vi "Read Waveform from TDMS (Scaled and Reduced Resolution).vi"(0 "VISA resource name":refnum<visa-resource-name>, 1 "Start Point (0)":i32, 2 "TDMS Path":path, 5 "Measurement Source (1: Channel 1)":i32(ring)=1 items=["Channel 1"=1, "Channel 2"=2, "Channel 3"=3, "Channel 4"=4, "Function 1"=5, "Function 2"=6, "Function 3"=7, "Function 4"=8, "Memory 1"=9, "Memory 2"=10, "Memory 3"=11, "Memory 4"=12], 7 "Length (1000)":i32=10000 caption="Length (10000)", 9 "Waveform Size (100)":i32=1000 caption="Waveform Size (1000)", 11 "error in (no error)":errorcluster) -> (4 "VISA resource name out":refnum<visa-resource-name>, 6 "Waveform Information":T1, 8 "Waveform Data":waveform(dbl)(graph), 15 "error out":errorcluster)   [LabVIEW 2020, in "Agilent 90000 Series.lvlib"]
doc: "Returns a decimated and scaled waveform. The points will be read from TDMS in chunks and a Min/Max decimating is performed on them."
uses:
  Agilent 90000 Series.lvlib
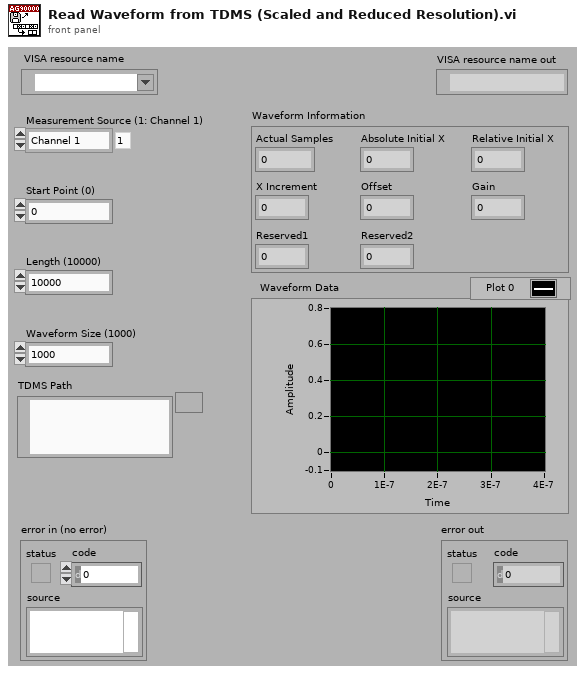
[diagram p1: front panel]
types:
  T1 = cluster{"Actual Samples":i32, "Absolute Initial X":dbl, "Relative Initial X":dbl, "X Increment":dbl, "Offset":dbl, "Gain":dbl, "Reserved1":dbl, "Reserved2":dbl}
  T2 = enum16{"open", "open or create", "create or replace", "create", "open (read-only)"}
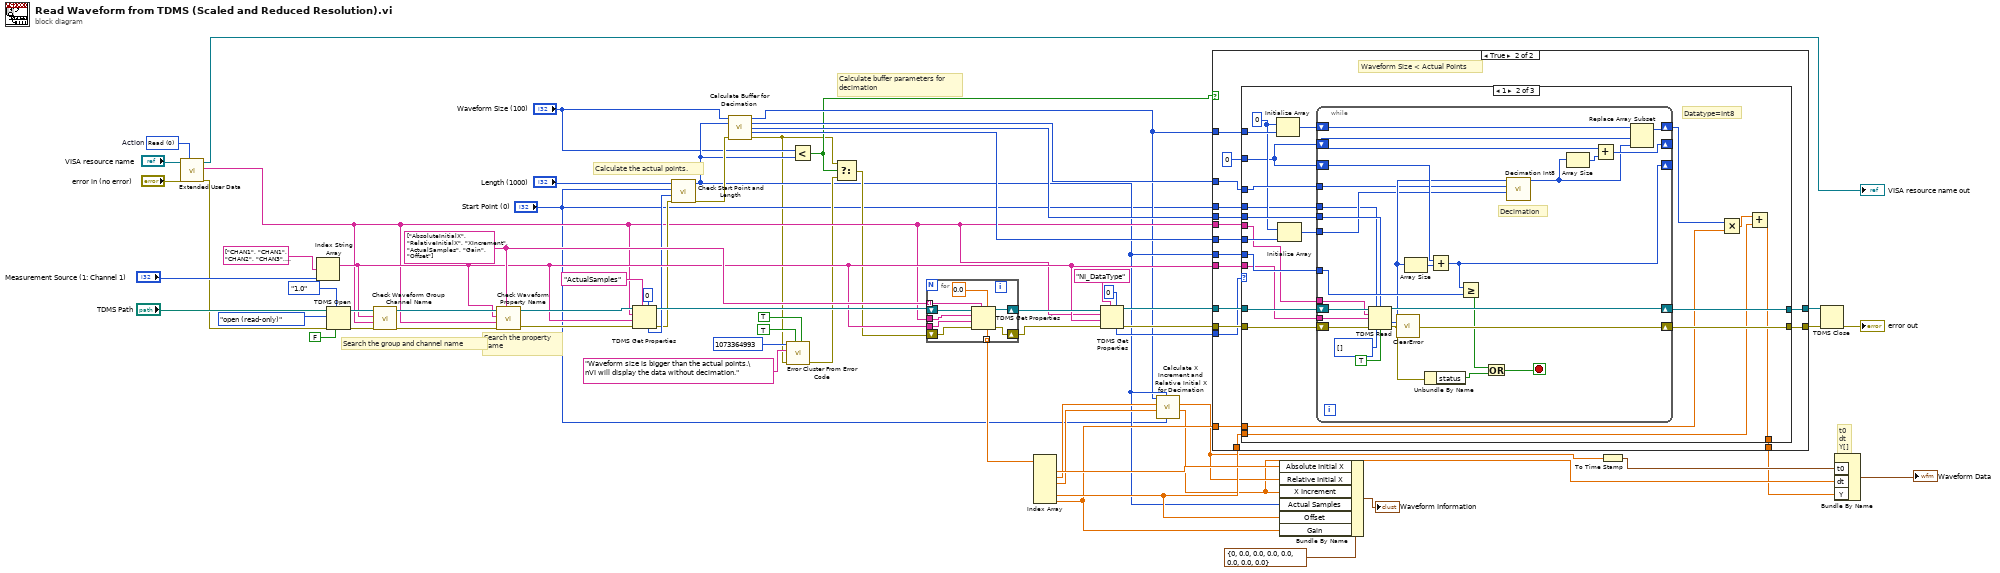
[diagram p0: block diagram]
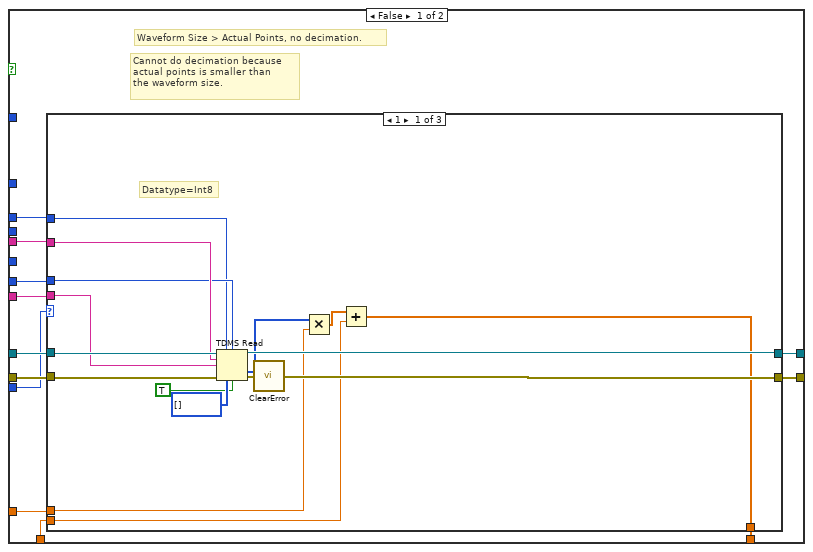
[diagram p2: hidden frame]
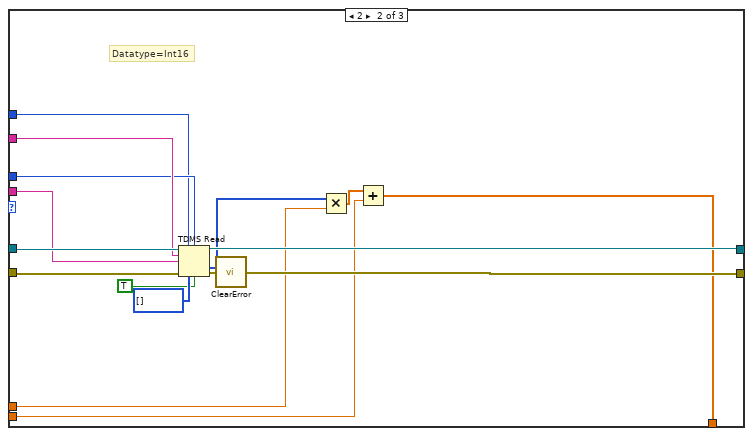
[diagram p3: hidden frame]
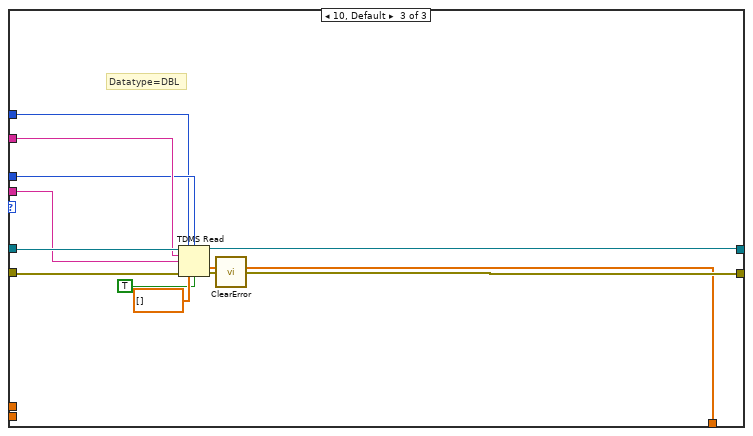
[diagram p4: hidden frame]
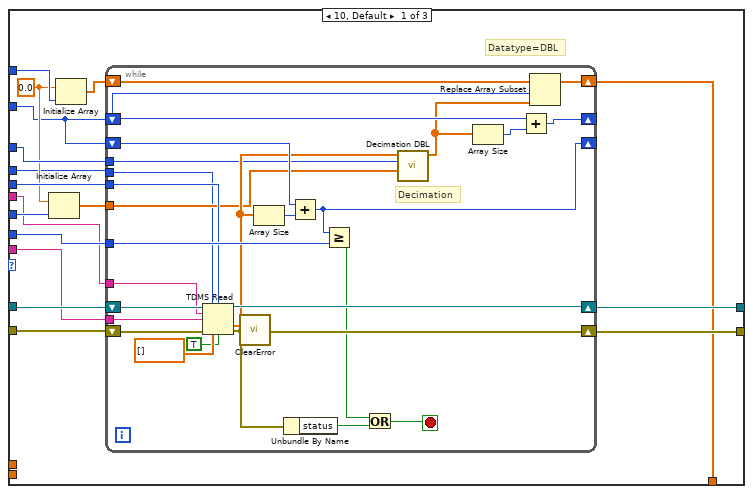
[diagram p5: hidden frame]
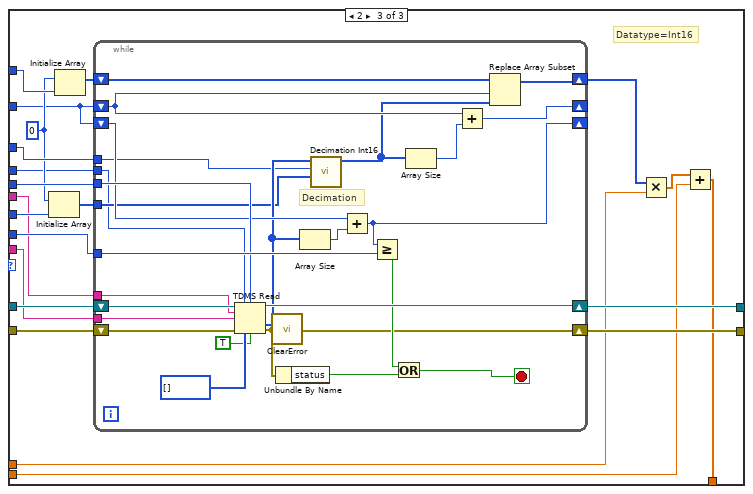
[diagram p6: hidden frame]
diagram:
  w26 = u16 0 items=["Read", "Write"]  # Action
  w57 = string[] ["AbsoluteInitialX", "RelativeInitialX", "XIncrement", "ActualSamples", "Gain", "Offset"] ("property names")
  # "t0\ndt\nY[]"
  # "Calculate buffer parameters for\ndecimation"
  # "Calculate the actual points."
  # "Search the property\nname"
  # "Search the group and channel name"
  n1 = call "Extended User Data.vi"("Action"=w26, "Error In (no error)"="error in (no error)", "VISA resource name in"="VISA resource name") -> ("Error Out"=w24:errorcluster, "Default Group Name Out"=w25:string, "VISA resource name out"=→"VISA resource name out":refnum<visa-resource-name>)  [unwired: 1 in, 5 out]
  n2 = Index String Array(1:"Measurement Source (1: Channel 1)", 2:string[] ["CHAN1", "CHAN1", "CHAN2", "CHAN3", "CHAN4", "FUNC1", "FUNC2", "FUNC3", "FUNC4", "WMEM1", "WMEM2", "WMEM3", "WMEM4"] ("subarray 2")) -> (0:w36:string)  [unwired: 1 out]
  n3 = TDMS Open(6:FALSE ("disable buffering? (T)"), 7:enum16{"1.0", "2.0"}."1.0" ("file format version (2.0)"), 8:w24, 10:T2."open (read-only)" ("operation (0:open)"), 11:"TDMS Path") -> (0:w55:errorcluster, 3:w56:refnum<k34>)  [unwired: 2 in]
  n4 = call "Check Waveform Group Channel Name.vi"("error in (no error)"=w55, "Group Name"=w25, "Channel Name"=w36, "TDMS File In"=w56) -> ("error out"=w54:errorcluster, "TDMS File Out"=w53:refnum<k34>)  [unwired: 6 out]
  n5 = call "Check Waveform Property Name.vi"("Property Name"=w57, "error in (no error)"=w54, "Group Name"=w25, "Channel Name"=w36, "TDMS File In"=w53) -> ("error out"=w50:errorcluster, "TDMS File Out"=w49:refnum<k34>)  [unwired: 5 out]
  n6 = TDMS Get Properties(5:0 ("Ring"), 7:"ActualSamples" ("property name"), 8:w50, 9:w36, 10:w25, 11:w49) -> (0:w31:errorcluster, 3:w46:refnum<k34>, 4:w32:i32)  [unwired: 3 out]
  n7 = call "Check Start Point and Length.vi"("error in (no error)"=w31, "Total Samples in TDMS (10000)"=w32, "Start Point (0)"="Start Point (0)", "Length (1000)"="Length (1000)") -> ("error out"=w30:errorcluster, "Actual Points"=w11:i32)  [unwired: 6 out]
  n8 = call "Calculate Buffer for Decimation.vi"("Waveform Size In (100)"="Waveform Size (100)", "Actual Points (1000)"=w11, "error in (no error)"=w30) -> ("Waveform Size Out"=w8:i32, "Number of Bytes per Chunck"=w10:i32, "Number of Bytes per Fetch"=w34:i32, "Decimation Buffer Size"=w33:i32, "error out"=w3:errorcluster)  [unwired: 1 in, 7 out]
  n9 = call <vilib>:"Error Cluster From Error Code.vi"("is warning? (False)"=TRUE, "show call chain? (False)"=TRUE, "error in (no error)"=w3, "error message (\"\")"="Waveform size is bigger than the actual points.\nVI will display the data without decimation." ("error message (\"\")"), "error code (0)"=1073364993) -> ("error out"=w20:errorcluster)  [unwired: 4 out]
  n10 = Less?(x="Waveform Size (100)", y=w11) -> (x < y?=w7:bool)
  n11 = Select(t=w3, s=w7, f=w20) -> (s? t:f=w19:errorcluster)
  n12 = for {
    tunnel: w36 -> [w71]
    tunnel: w25 -> [w70]
    shift-right: [w72] -> w42
    shift-left: w19 -> [w73]
    tunnel: w57 -> [w68] mode=indexing
    tunnel: [w66] -> w61 mode=indexing
    shift-right: [w69] -> w45
    shift-left: w46 -> [w74]
    n13 = TDMS Get Properties(5:0.0 ("Reserved1"), 7:w68, 8:w73, 9:w71, 10:w70, 11:w74) -> (0:w72:errorcluster, 3:w69:refnum<k34>, 4:w66:dbl)  [unwired: 3 out]
  }
  n14 = Index Array(array=w61) -> (element #1=w60:dbl, element #2=w18:dbl, element #3=w17:dbl, element #5=w40:dbl, element #6=w39:dbl)  [unwired: 6 in, 1 out]
  n15 = TDMS Get Properties(5:0 ("Ring"), 7:"NI_DataType" ("property name"), 8:w42, 9:w36, 10:w25, 11:w45) -> (0:w43:errorcluster, 3:w44:refnum<k34>, 4:w41:i32)  [unwired: 3 out]
  n16 = call "Calculate X Increment and Relative Initial X for Decimation.vi"("Start Point (0)"="Start Point (0)", "Actual Points (1000)"=w11, "Original X Increment (0)"=w17, "Original Relative Initial X (0)"=w18, "Waveform Size (100)"=w8) -> ("X Increment Out"=w13:dbl, "Relative Initial X Out"=w15:dbl)  [unwired: 5 out]
  n17 = case shown="True" w7 {
    tunnel: w44 -> [w86 w147]
    tunnel: w43 -> [w85 w146]
    tunnel: w41 -> [w84 w145]
    tunnel: w40 -> [w83 w144]
    tunnel: w39 -> [w82 w143]
    tunnel: [w81 w142] -> w38
    tunnel: [w80 w141] -> w37
    tunnel: w36 -> [w79 w140]
    tunnel: w34 -> [_ w139]
    tunnel: w33 -> [_ w138]
    tunnel: w25 -> [w78 w137]
    tunnel: [w77 w135] -> w5
    tunnel: w11 -> [w76 w134]
    tunnel: w10 -> [_ w133]
    tunnel: w8 -> [_ w132]
    tunnel: "Start Point (0)" -> [w75 w131]
    frame False {
      # "Cannot do decimation because\nactual points is smaller than \nthe waveform size."
      # "Waveform Size > Actual Points, no decimation."
      n18 = case shown="1" w84 {
        tunnel: w78 -> [w100 w116 w128]
        tunnel: w79 -> [w99 w115 w127]
        tunnel: w86 -> [w101 w117 w129]
        tunnel: w85 -> [w102 w118 w130]
        tunnel: w83 -> [w95 w111 _]
        tunnel: w82 -> [w96 w112 _]
        tunnel: w76 -> [w92 w108 w123]
        tunnel: [w98 w114 w126] -> w81
        tunnel: [w97 w113 w125] -> w80
        tunnel: [w89 w105 w121] -> w77
        tunnel: w75 -> [w91 w107 w122]
        frame 1 {
          # "Datatype=Int8"
          n19 = TDMS Read(0:w101, 1:w91, 2:w92, 5:w100, 7:w99, 11:w102, 12:i8[] [], 13:TRUE ("return channels in file order? (F)")) -> (4:w98:refnum<k34>, 10:w90:i8[], 15:w87:errorcluster)  [unwired: 3 out]
          n20 = call <vilib>:"ClearError.vi"("error in (no error)"=w87) -> ("error out"=w97:errorcluster)
          n21 = Multiply(x=w90, y=w96) -> (x*y=w94:dbl[])
          n22 = Add(x=w94, y=w95) -> (x+y=w89:dbl[])
        }
        frame 2 {
          # "Datatype=Int16"
          n23 = TDMS Read(0:w117, 1:w107, 2:w108, 5:w116, 7:w115, 11:w118, 12:i16[] [], 13:TRUE ("return channels in file order? (F)")) -> (4:w114:refnum<k34>, 10:w106:i16[], 15:w103:errorcluster)  [unwired: 3 out]
          n24 = call <vilib>:"ClearError.vi"("error in (no error)"=w103) -> ("error out"=w113:errorcluster)
          n25 = Multiply(x=w106, y=w112) -> (x*y=w110:dbl[])
          n26 = Add(x=w110, y=w111) -> (x+y=w105:dbl[])
        }
        frame 10, Default {
          # "Datatype=DBL"
          n27 = TDMS Read(0:w129, 1:w122, 2:w123, 5:w128, 7:w127, 11:w130, 12:dbl[] [], 13:TRUE ("return channels in file order? (F)")) -> (4:w126:refnum<k34>, 10:w121:dbl[], 15:w119:errorcluster)  [unwired: 3 out]
          n28 = call <vilib>:"ClearError.vi"("error in (no error)"=w119) -> ("error out"=w125:errorcluster)
        }
      }
    }
    frame True {
      # "Waveform Size < Actual Points"
      n29 = case shown="1" w145 {
        tunnel: w137 -> [w154 w202 w250]
        tunnel: w140 -> [w153 w201 w249]
        tunnel: w147 -> [w155 w203 w251]
        tunnel: w146 -> [w156 w204 w252]
        tunnel: w144 -> [_ w194 w242]
        tunnel: w143 -> [_ w197 w245]
        tunnel: w132 -> [w164 w212 w260]
        tunnel: 0 ("element") -> [w149 w195 w243]
        tunnel: w133 -> [w162 w210 w258]
        tunnel: w139 -> [w161 w209 w257]
        tunnel: w138 -> [w159 w207 w255]
        tunnel: w134 -> [w157 w205 w253]
        tunnel: [w152 w200 w248] -> w142
        tunnel: [w151 w199 w247] -> w141
        tunnel: [w150 w196 w244] -> w135
        tunnel: w131 -> [w148 w192 w240]
        frame 10, Default {
          w160 = 0.0 ("element")
          # "Datatype=DBL"
          n30 = Initialize Array(w160, w159) -> (w158:dbl[])
          n31 = Initialize Array(w160, w164) -> (w163:dbl[])
          n32 = while {
            shift-right: [w175] -> w151
            shift-left: w156 -> [w182]
            shift-right: [w191] -> w152
            shift-left: w155 -> [w190]
            shift-right: [w189] -> w150
            shift-left: w163 -> [w187]
            shift-right: [w188] -> _
            shift-left: w149 -> [w176]
            tunnel: w157 -> [w186]
            tunnel: w161 -> [w179]
            tunnel: w162 -> [w170]
            tunnel: w158 -> [w169]
            shift-right: [w183] -> _
            shift-left: w149 -> [w185]
            tunnel: w154 -> [w178]
            tunnel: w153 -> [w177]
            tunnel: w148 -> [w167]
            stop <- w172 stop-if-true
            # "Decimation"
            n33 = TDMS Read(0:w190, 1:w167, 2:w179, 5:w178, 7:w177, 11:w182, 12:dbl[] [], 13:TRUE ("return channels in file order? (F)")) -> (4:w191:refnum<k34>, 10:w171:dbl[], 15:w165:errorcluster)  [unwired: 3 out]
            n34 = call <vilib>:"ClearError.vi"("error in (no error)"=w165) -> ("error out"=w175:errorcluster)
            n35 = Array Size(array=w171) -> (size(s)=w180:i32)
            n36 = Unbundle By Name(w175) -> ("status"=w174:bool)
            n37 = Add(x=w176, y=w180) -> (x+y=w188:i32)
            n38 = Greater Or Equal?(x=w188, y=w186) -> (x >= y?=w173:bool)
            n39 = Or(x=w173, y=w174) -> (x .or. y?=w172:bool)
            n40 = call "Decimation DBL.vi"("Decimation Array"=w169, "Number of Bytes per Chunck (1000)"=w170, "Raw Data"=w171) -> ("Decimation Data"=w168:dbl[])  [unwired: 8 out]
            n41 = Array Size(array=w168) -> (size(s)=w184:i32)
            n42 = Add(x=w185, y=w184) -> (x+y=w183:i32)
            n43 = Replace Array Subset(array=w187, new element=w168, index=w185) -> (w189:dbl[])
          }
        }
        frame 1 {
          w208 = i8 0 ("element")
          # "Datatype=Int8"
          n44 = Initialize Array(w208, w212) -> (w211:i8[])
          n45 = Initialize Array(w208, w207) -> (w206:i8[])
          n46 = while {
            shift-right: [w222] -> w199
            shift-left: w204 -> [w230]
            shift-right: [w239] -> w200
            shift-left: w203 -> [w238]
            shift-right: [w237] -> w198
            shift-left: w211 -> [w235]
            shift-right: [w236] -> _
            shift-left: w195 -> [w224]
            tunnel: w205 -> [w234]
            tunnel: w209 -> [w227]
            tunnel: w210 -> [w218]
            tunnel: w206 -> [w217]
            shift-right: [w231] -> _
            shift-left: w195 -> [w233]
            tunnel: w202 -> [w226]
            tunnel: w201 -> [w225]
            tunnel: w192 -> [w215]
            stop <- w220 stop-if-true
            # "Decimation"
            n47 = TDMS Read(0:w238, 1:w215, 2:w227, 5:w226, 7:w225, 11:w230, 12:i8[] [], 13:TRUE ("return channels in file order? (F)")) -> (4:w239:refnum<k34>, 10:w219:i8[], 15:w213:errorcluster)  [unwired: 3 out]
            n48 = call <vilib>:"ClearError.vi"("error in (no error)"=w213) -> ("error out"=w222:errorcluster)
            n49 = Array Size(array=w219) -> (size(s)=w228:i32)
            n50 = Unbundle By Name(w222) -> ("status"=w223:bool)
            n51 = Add(x=w224, y=w228) -> (x+y=w236:i32)
            n52 = Greater Or Equal?(x=w236, y=w234) -> (x >= y?=w221:bool)
            n53 = Or(x=w221, y=w223) -> (x .or. y?=w220:bool)
            n54 = call "Decimation Int8.vi"("Decimation Array"=w217, "Number of Bytes per Chunck (1000)"=w218, "Raw Data"=w219) -> ("Decimation Data"=w216:i8[])  [unwired: 8 out]
            n55 = Array Size(array=w216) -> (size(s)=w232:i32)
            n56 = Add(x=w233, y=w232) -> (x+y=w231:i32)
            n57 = Replace Array Subset(array=w235, new element=w216, index=w233) -> (w237:i8[])
          }
          n58 = Multiply(x=w198, y=w197) -> (x*y=w193:dbl[])
          n59 = Add(x=w193, y=w194) -> (x+y=w196:dbl[])
        }
        frame 2 {
          w256 = i16 0 ("element")
          # "Datatype=Int16"
          n60 = Initialize Array(w256, w255) -> (w254:i16[])
          n61 = Initialize Array(w256, w260) -> (w259:i16[])
          n62 = while {
            shift-right: [w268] -> w247
            shift-left: w252 -> [w278]
            shift-right: [w287] -> w248
            shift-left: w251 -> [w286]
            shift-right: [w285] -> w246
            shift-left: w259 -> [w283]
            shift-right: [w284] -> _
            shift-left: w243 -> [w272]
            tunnel: w253 -> [w282]
            tunnel: w257 -> [w275]
            tunnel: w258 -> [w266]
            tunnel: w254 -> [w265]
            shift-right: [w279] -> _
            shift-left: w243 -> [w281]
            tunnel: w250 -> [w274]
            tunnel: w249 -> [w273]
            tunnel: w240 -> [w263]
            stop <- w270 stop-if-true
            # "Decimation"
            n63 = TDMS Read(0:w286, 1:w263, 2:w275, 5:w274, 7:w273, 11:w278, 12:i16[] [], 13:TRUE ("return channels in file order? (F)")) -> (4:w287:refnum<k34>, 10:w267:i16[], 15:w261:errorcluster)  [unwired: 3 out]
            n64 = call <vilib>:"ClearError.vi"("error in (no error)"=w261) -> ("error out"=w268:errorcluster)
            n65 = Unbundle By Name(w268) -> ("status"=w271:bool)
            n66 = Array Size(array=w267) -> (size(s)=w276:i32)
            n67 = call "Decimation Int16.vi"("Decimation Array"=w265, "Number of Bytes per Chunck (1000)"=w266, "Raw Data"=w267) -> ("Decimation Data"=w264:i16[])  [unwired: 8 out]
            n68 = Add(x=w272, y=w276) -> (x+y=w284:i32)
            n69 = Greater Or Equal?(x=w284, y=w282) -> (x >= y?=w269:bool)
            n70 = Or(x=w269, y=w271) -> (x .or. y?=w270:bool)
            n71 = Array Size(array=w264) -> (size(s)=w280:i32)
            n72 = Add(x=w281, y=w280) -> (x+y=w279:i32)
            n73 = Replace Array Subset(array=w283, new element=w264, index=w281) -> (w285:i16[])
          }
          n74 = Multiply(x=w246, y=w245) -> (x*y=w241:dbl[])
          n75 = Add(x=w241, y=w242) -> (x+y=w244:dbl[])
        }
      }
    }
  }
  n76 = Bundle By Name(cluster=T1 {"Actual Samples"=0, "Absolute Initial X"=0.0, "Relative Initial X"=0.0, "X Increment"=0.0, "Offset"=0.0, "Gain"=0.0, "Reserved1"=0.0, "Reserved2"=0.0} ("Waveform Information"), "Absolute Initial X"=w60, "Relative Initial X"=w15, "X Increment"=w13, "Actual Samples"=w11, "Offset"=w40, "Gain"=w39) -> (→"Waveform Information":T1)
  n77 = To Time Stamp(1:w15) -> (0:w14:timestamp)
  n78 = TDMS Close(8:w37, 11:w38) -> (0:→"error out":errorcluster)  [unwired: 1 out]
  n79 = Bundle By Name ("Build Waveform")("t0"=w14, "dt"=w13, "Y"=w5) -> (→"Waveform Data":waveform(dbl))  [unwired: 1 out]
